vi "Sort 1D Array with Sort Order output.vi"(2 "Disordered Array":dbl[](array[numeric]), 3 "Sort Order":enum16{"Ascending", "Descending"}(ring)) -> (0 "Ordered Array":dbl[](array[numeric]), 1 "Original Indices":i32[](array[numeric]))   [LabVIEW 2015]
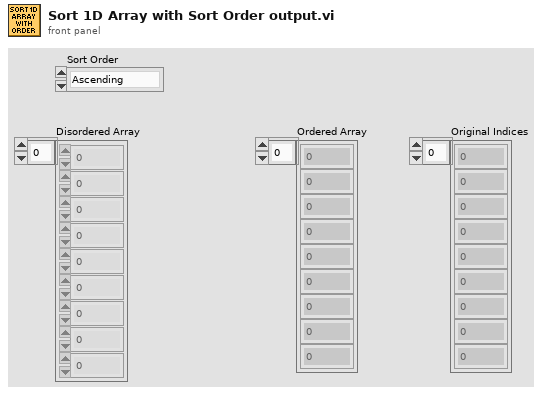
[diagram p1: front panel]
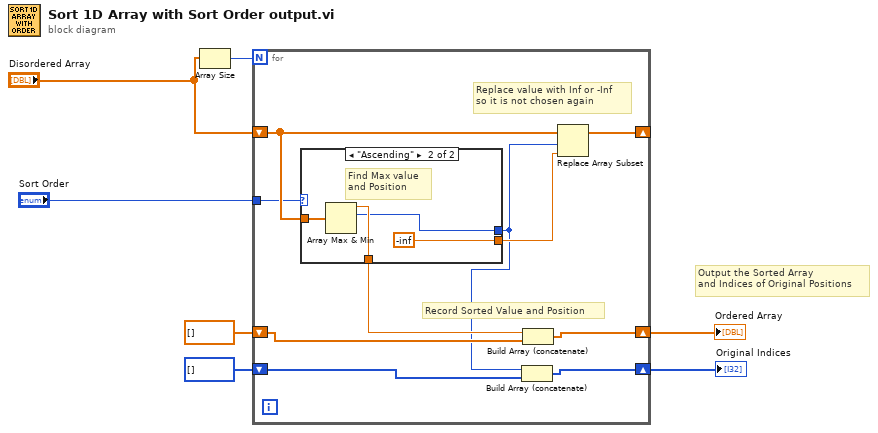
[diagram p0: block diagram]
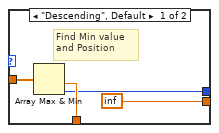
[diagram p2: hidden frame]
diagram:
  # "Output the Sorted Array\nand Indices of Original Positions"
  n1 = Array Size(array="Disordered Array") -> (size(s)=w7:i32)
  n2 = for {
    N: w7 -> [_]
    shift-right: [w13] -> _
    shift-left: "Disordered Array" -> [w15]
    shift-right: [w17] -> w6
    shift-left: dbl[] [] -> [w10]
    shift-right: [w16] -> w5
    shift-left: i32[] [] -> [w9]
    tunnel: "Sort Order" -> [w12]
    # "Record Sorted Value and Position"
    # "Replace value with Inf or -Inf \nso it is not chosen again"
    n3 = case shown="\"Ascending\"" w12 {
      tunnel: [w21 w23] -> w11
      tunnel: w15 -> [w20 w25]
      tunnel: [inf -inf] -> w14
      tunnel: [w18 w22] -> w8
      frame "Descending", Default {
        # "Find Min value \nand Position"
        n4 = Array Max & Min(array=w20) -> (min value=w21:dbl, min index (indices)=w18:i32)  [unwired: 2 out]
      }
      frame "Ascending" {
        # "Find Max value \nand Position"
        n5 = Array Max & Min(array=w25) -> (max value=w23:dbl, max index (indices)=w22:i32)  [unwired: 2 out]
      }
    }
    n6 = Build Array (concatenate)(w8, w9) -> (w16:i32[])
    n7 = Build Array (concatenate)(w11, w10) -> (w17:dbl[])
    n8 = Replace Array Subset(array=w15, new element=w14, index=w8) -> (w13:dbl[])
  }
  "Ordered Array" <- w6
  "Original Indices" <- w5
